vi "Error Handler.vi"(6 "errlog Name":string="Errors.log", 7 "Module":string, 8 "error in (no error)":errorcluster, 9 "Enable LogFile?(T)":bool=TRUE) -> (0 "error out":errorcluster)   [LabVIEW 2017, in "Error Handler.lvlib"]
uses:
  Error Handler.lvlib
  Def-ModuleError--Cluster.ctl
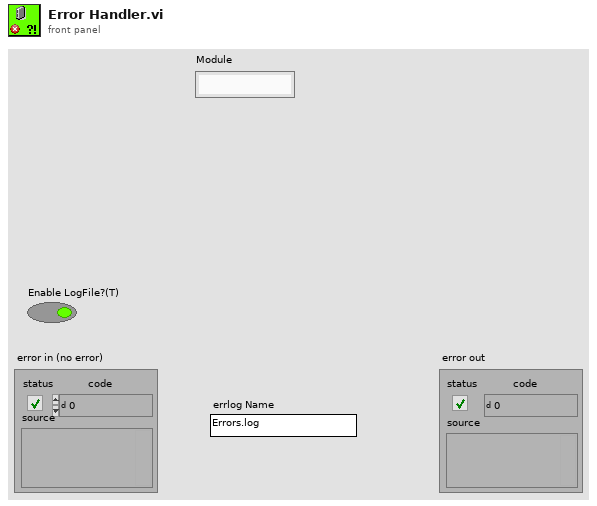
[diagram p1: front panel]
types:
  T1 = typedef "Error Handler.lvlib/Def-ModuleError--Cluster.ctl" = cluster{"Module":string, "error":errorcluster}
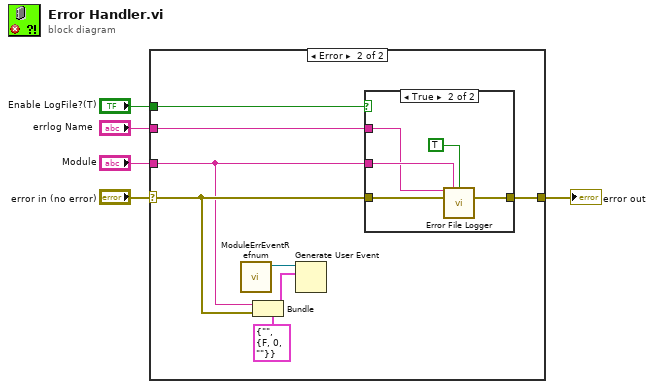
[diagram p0: block diagram]
diagram:
  n1 = case shown="Error" "error in (no error)" {
    selector: "error in (no error)" -> [w6 w11]
    tunnel: [w6 w14] -> w4
    tunnel: "Module" -> [_ w9]
    tunnel: "errlog Name" -> [_ w8]
    tunnel: "Enable LogFile?(T)" -> [_ w7]
    frame No Error {
    }
    frame Error {
      n2 = call "ModuleErrEventRefnum.vi"() -> ("ModuleError"=w13:refnum<user-event>)  [unwired: 9 in, 2 out]
      n3 = Bundle(cluster=T1 {"Module"="", "error"={"status"=FALSE, "code"=0, "source"=""}} ("ModuleError--Cluster"), "Module"=w9, "error"=w11) -> (w12:T1)
      n4 = Generate User Event(user event=w13, event data cluster=w12) -> ()  [unwired: 2 in, 2 out]
      n5 = case shown="True" w7 {
        tunnel: [w15 w20] -> w14
        tunnel: w11 -> [w15 w18]
        tunnel: w9 -> [_ w17]
        tunnel: w8 -> [_ w16]
        frame False {
        }
        frame True {
          n6 = call "Error File Logger.vi"("errlog Name"=w16, "Module"=w17, "Clear Error?"=TRUE, "error in (no error)"=w18) -> ("error out"=w20:errorcluster)  [unwired: 10 in, 1 out]
        }
      }
    }
  }
  "error out" <- w4
